vi "Restore Waveform Array.vi"(0 "waveform t0 array":dbl[](array[numeric]), 5 "waveform dt array":dbl[](array[numeric]), 7 "waveform length array":i32[](array[numeric]), 9 "concatenated waveform Y":dbl[](array[numeric])) -> (4 "waveform array":waveform(dbl)[](array[waveform]))   [LabVIEW 2021, in "PMIC Common.lvlib"]
uses:
  PMIC Common.lvlib
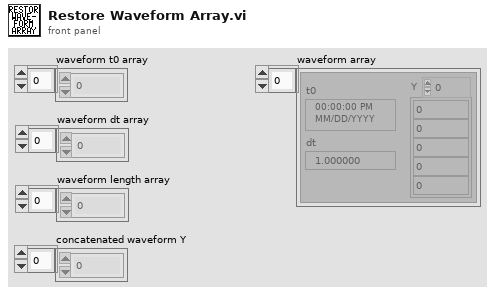
[diagram p1: front panel]
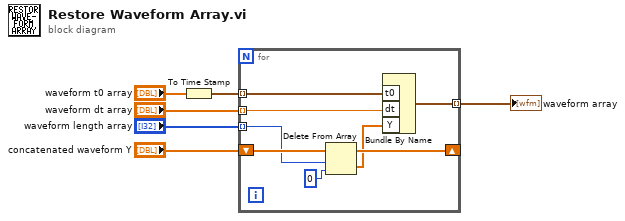
[diagram p0: block diagram]
diagram:
  n1 = To Time Stamp(1:"waveform t0 array") -> (0:w5:timestamp[])
  n2 = for {
    tunnel: w5 -> [w11] mode=indexing
    tunnel: "waveform dt array" -> [w10] mode=indexing
    shift-right: [w12] -> _
    shift-left: "concatenated waveform Y" -> [w14]
    tunnel: "waveform length array" -> [w13] mode=indexing
    tunnel: [w8] -> w1 mode=indexing
    n3 = Delete From Array(array=w14, length=w13, index=0) -> (deleted portion=w9:dbl[], array with subset deleted=w12:dbl[])
    n4 = Bundle By Name("t0"=w11, "dt"=w10, "Y"=w9) -> (w8:waveform(dbl))  [unwired: 1 in]
  }
  "waveform array" <- w1
